vi "Notify_User.vi"(0 "Last_Error_Details":T1 caption="Last Error Details", 11 "Error_In":errorcluster) -> (4 "Exit?":bool, 15 "Error_Out":errorcluster)   [LabVIEW 2023]
doc: "Notify user is used to notify the user about the Error."
uses:
  Last_Error_Details.ctl
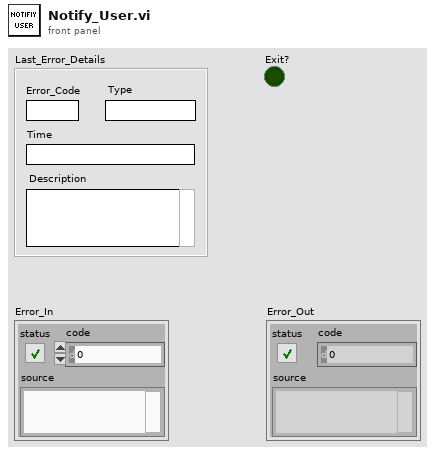
[diagram p1: front panel]
types:
  T1 = typedef "Last_Error_Details.ctl" = cluster{"Error_Code":string, "Type":string, "Time":string, "Description":string}
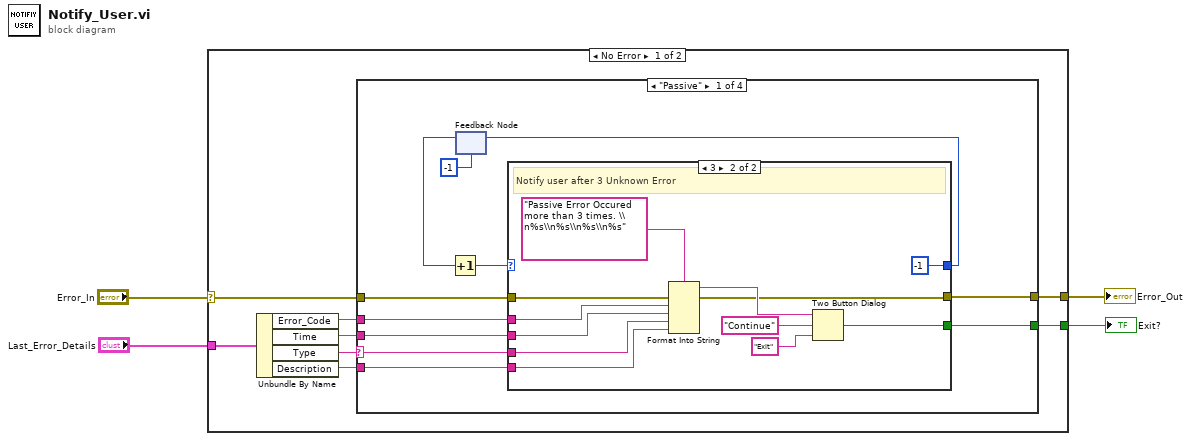
[diagram p0: block diagram]
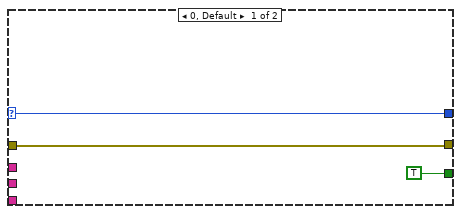
[diagram p2: hidden frame]
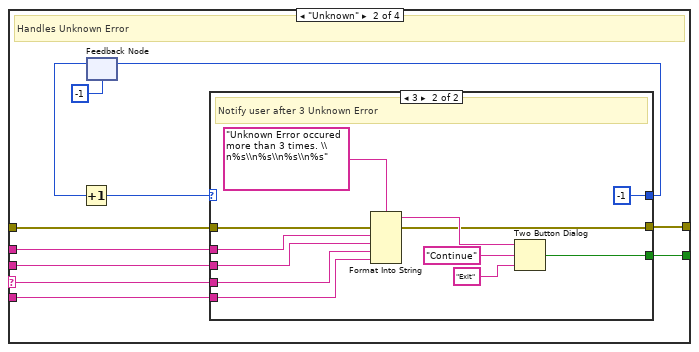
[diagram p3: hidden frame]
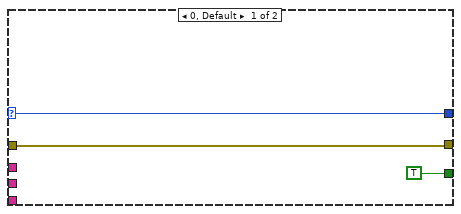
[diagram p4: hidden frame]
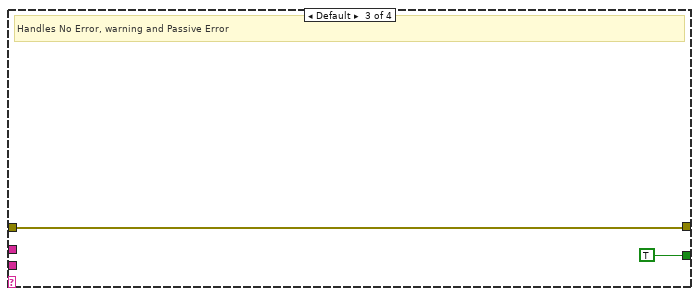
[diagram p5: hidden frame]
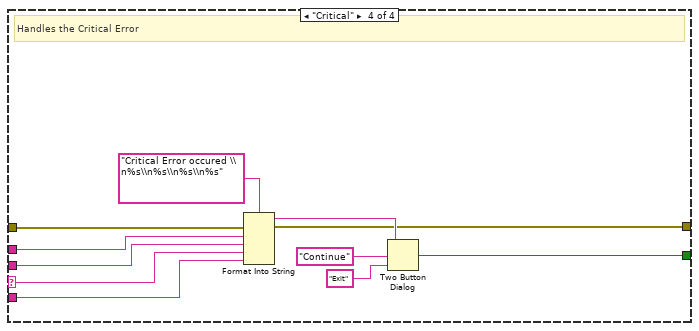
[diagram p6: hidden frame]
diagram:
  n1 = case shown="No Error" "Error_In" {
    selector: "Error_In" -> [w6 w78]
    tunnel: "Last_Error_Details" -> [w8 _]
    tunnel: [w7 _] -> w3
    tunnel: [w5 w78] -> w1
    frame No Error {
      n2 = Unbundle By Name(w8) -> ("Error_Code"=w12:string, "Time"=w9:string, "Type"=w10:string, "Description"=w11:string)
      n3 = case shown="\"Passive\"" w10 {
        selector: w10 -> [w16 w48 _ w75]
        tunnel: w12 -> [w18 w46 _ w76]
        tunnel: w11 -> [w15 w49 _ w74]
        tunnel: w9 -> [w17 w47 _ w73]
        tunnel: [w13 w41 TRUE ("T button?") w69] -> w7
        tunnel: w6 -> [w19 w40 w65 w68]
        tunnel: [w14 w39 w65 w67] -> w5
        frame "Passive" {
          n4 = feedback #1(-1) -> (w21:i32)
          n5 = Increment(x=w21) -> (x+1=w22:i32)
          n6 = case shown="3" w22 {
            selector: w22 -> [w26 _]
            tunnel: w15 -> [_ w34]
            tunnel: w16 -> [_ w33]
            tunnel: w17 -> [_ w32]
            tunnel: w18 -> [_ w31]
            tunnel: [w26 -1] -> w20
            tunnel: [TRUE w29] -> w13
            tunnel: w19 -> [w24 w28]
            tunnel: [w24 w27] -> w14
            frame 0, Default {
            }
            frame 3 {
              # "Notify user after 3 Unknown Error"
              n7 = Format Into String(format string="Passive Error Occured more than 3 times. \\n%s\\n%s\\n%s\\n%s", error in=w28, w31, w32, w33, w34) -> (resulting string=w37:string, error out=w27:errorcluster)  [unwired: 1 in]
              n8 = Two Button Dialog(message=w37, 1:"Exit" ("F button name (\"Cancel\")"), 2:"Continue" ("T button name (\"OK\")")) -> (T button?=w29:bool)
            }
          }
          n9 = feedback-in #1(w20) -> ()
        }
        frame "Unknown" {
          # "Handles Unknown Error"
          n10 = feedback #2(-1) -> (w43:i32)
          n11 = Increment(x=w43) -> (x+1=w44:i32)
          n12 = case shown="3" w44 {
            selector: w44 -> [w52 _]
            tunnel: w49 -> [_ w60]
            tunnel: w48 -> [_ w59]
            tunnel: w47 -> [_ w58]
            tunnel: w46 -> [_ w57]
            tunnel: [w52 -1] -> w42
            tunnel: [TRUE w55] -> w41
            tunnel: w40 -> [w50 w54]
            tunnel: [w50 w53] -> w39
            frame 0, Default {
            }
            frame 3 {
              # "Notify user after 3 Unknown Error"
              n13 = Format Into String(format string="Unknown Error occured more than 3 times. \\n%s\\n%s\\n%s\\n%s", error in=w54, w57, w58, w59, w60) -> (resulting string=w63:string, error out=w53:errorcluster)  [unwired: 1 in]
              n14 = Two Button Dialog(message=w63, 1:"Exit" ("F button name (\"Cancel\")"), 2:"Continue" ("T button name (\"OK\")")) -> (T button?=w55:bool)
            }
          }
          n15 = feedback-in #2(w42) -> ()
        }
        frame Default {
          # "Handles No Error, warning and Passive Error"
        }
        frame "Critical" {
          # "Handles the Critical Error"
          n16 = Format Into String(format string="Critical Error occured \\n%s\\n%s\\n%s\\n%s", error in=w68, w76, w73, w75, w74) -> (resulting string=w72:string, error out=w67:errorcluster)  [unwired: 1 in]
          n17 = Two Button Dialog(message=w72, 1:"Exit" ("F button name (\"Cancel\")"), 2:"Continue" ("T button name (\"OK\")")) -> (T button?=w69:bool)
        }
      }
    }
    frame Error {
    }
  }
  "Exit?" <- w3
  "Error_Out" <- w1
